vi "niFPGA Matrix-Vector Product.vi"(11 "Vector b":fxp<+/-,16,8>[](array[numeric])=[0.0, 0.0, 0.0, 0.0, 0.0]) -> (3 "Vector c":fxp<+/-,35,19>[](array[numeric]))   [LabVIEW 2017]
doc: "Multiplies <B>Matrix A</B> by an input <B>Vector b</B>. This operation is useful for FPGA control applications, such as state-feedback control. You can use more than one multiplier to reduce the latency of this operation. To define <B>Matrix A</B>, double-click this Express VI and use the <B>Matrix Data Initialization</B> page to specify a VI, TXT, or CSV file that contains the matrix data. If you do not define <B>Matrix A</B>, this Express VI uses a matrix of zeroes instead."
uses:
  <vilib>/fxp/LVFixedPointOverflowPolicyTypeDef.ctl
  <vilib>/fxp/LVFixedPointQuantizationPolicyTypeDef.ctl
  <vilib>/rvi/Analysis/control/MatrixVector/Matrix Vector subs/niFPGAMatrixVector_TargetState.ctl
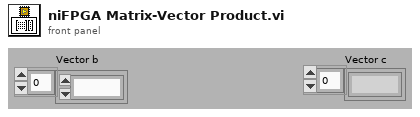
[diagram p1: front panel]
types:
  T1 = typedef "niFPGAMatrixVector_TargetState.ctl" = cluster{"matrix datatype":cluster{"sign?":bool, "word length":i32, "integer word length":i32}, "vector datatype":cluster{"sign?":bool, "word length":i32, "integer word length":i32}, "result datatype":cluster{"sign?":bool, "word length":i32, "integer word length":i32}, "matrix size":cluster{"matrix rows":i32, "matrix columns":i32}, "Adapt to source":bool, "Matrix A constant?":bool, "# multipliers":i32, "# number of multiplier pipeline":i32, "Overflow mode":T2, "Rounding mode":T3, "Initialization method":u16, "File path conversion":path, "Matrix data":ext[][], "Code generated":bool}
  T2 = typedef "LVFixedPointOverflowPolicyTypeDef.ctl" = enum32{"Wrap", "Saturate"}
  T3 = typedef "LVFixedPointQuantizationPolicyTypeDef.ctl" = enum32{"Truncate", "Round-Half-Up (Asymmetric)", "Round-Half-Even"}
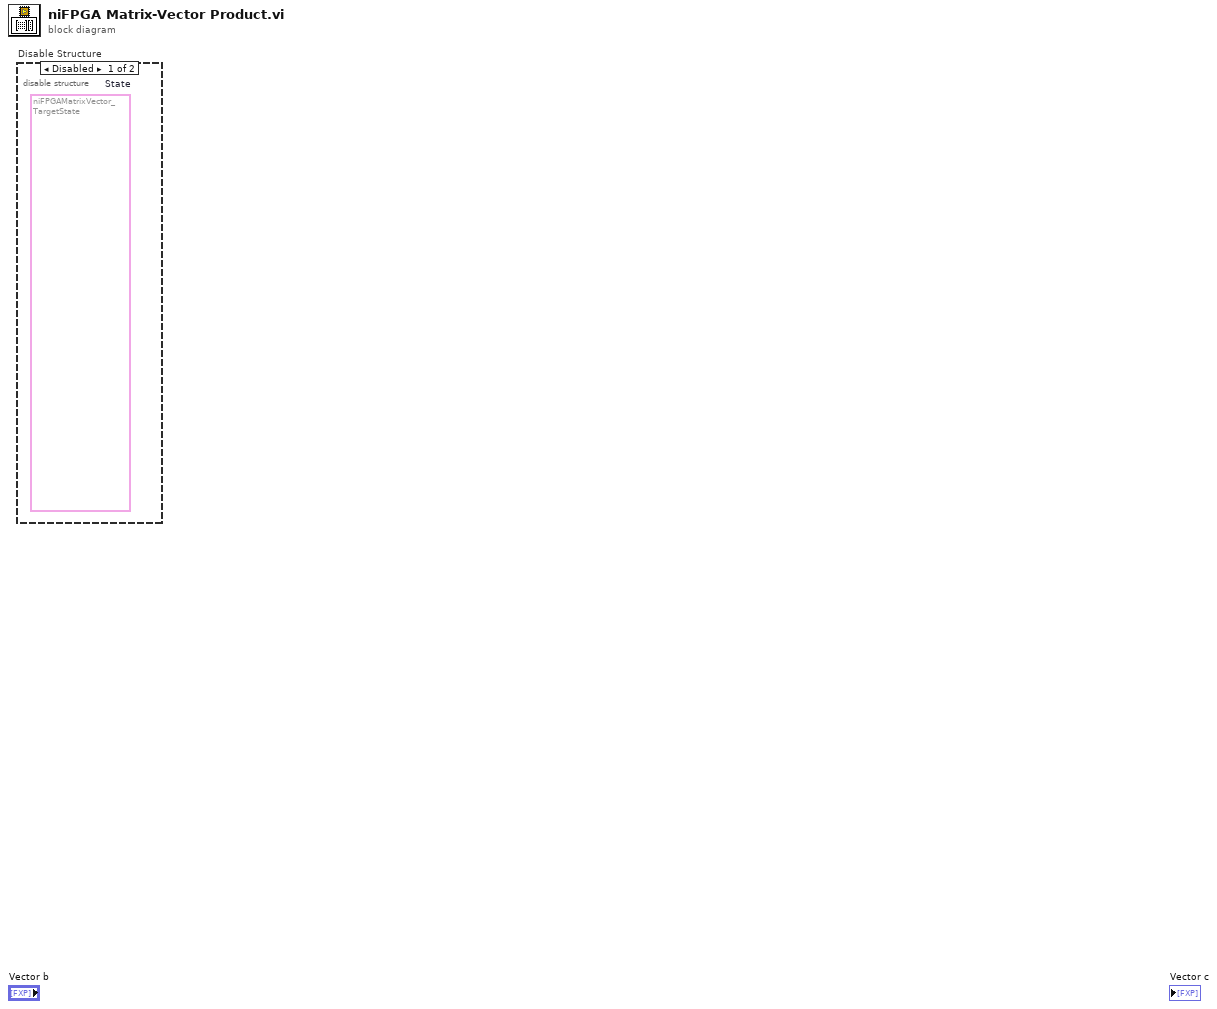
[diagram p0: block diagram]
diagram:
  n1 = disable-structure "Disable Structure" shown="Disabled" {
    frame Disabled {
      (unwired) T1 {"matrix datatype"={"sign?"=TRUE, "word length"=16, "integer word length"=8}, "vector datatype"={"sign?"=TRUE, "word length"=16, "integer word length"=8}, "result datatype"={"sign?"=TRUE, "word length"=35, "integer word length"=19}, "matrix size"={"matrix rows"=5, "matrix columns"=5}, "Adapt to source"=TRUE, "Matrix A constant?"=TRUE, "# multipliers"=1, "# number of multiplier pipeline"=0, "Overflow mode"=enum."Wrap", "Rounding mode"=enum."Truncate", "Initialization method"=0, "File path conversion"=path "", "Matrix data"=[[0.0, 0.0, 0.0, 0.0, 0.0], [0.0, 0.0, 0.0, 0.0, 0.0], [0.0, 0.0, 0.0, 0.0, 0.0], [0.0, 0.0, 0.0, 0.0, 0.0], [0.0, 0.0, 0.0, 0.0, 0.0]], "Code generated"=FALSE}  # State
    }
    frame Enabled {
    }
  }
